vi "M-686 Test Panel.vi"() -> ()   [LabVIEW 2020]
uses:
  <vilib>/Instr/_visa.llb/VISA Configure Serial Port (Instr).vi
panel:
  in  "Wait for Reply":bool=TRUE
  out "Bool":bool
  out "Value":dbl
  out "Cmd Success":bool
  out "Connected":bool
  out "Waiting for Reply":bool
  out "Last Error":errorcluster
  out "Command History":string
  out "Reply":string
  in  "Command":string
  in  "Quit":bool
  in  "COM Port":refnum<visa-resource-name>="COM4"
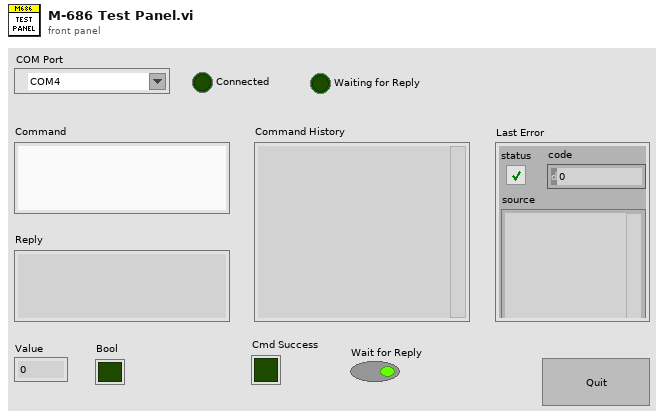
[diagram p1: front panel]
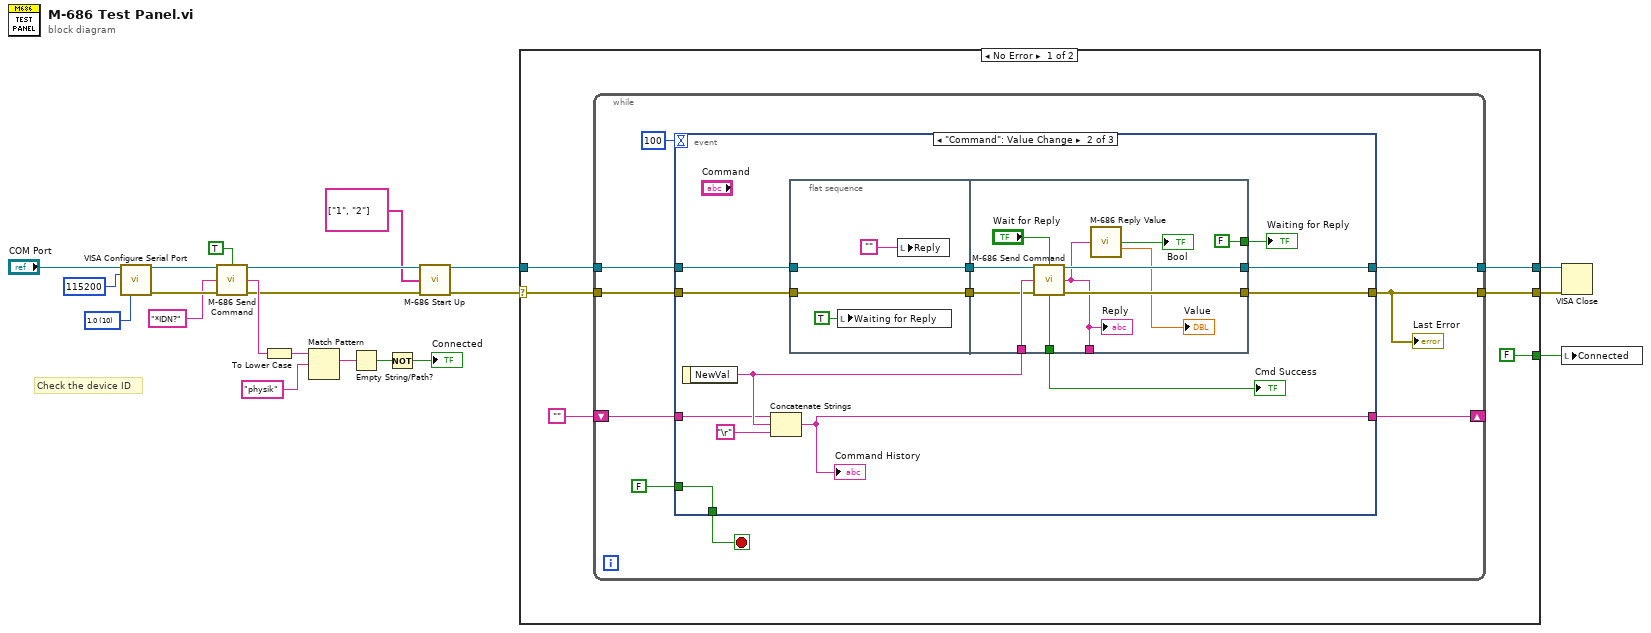
[diagram p0: block diagram]
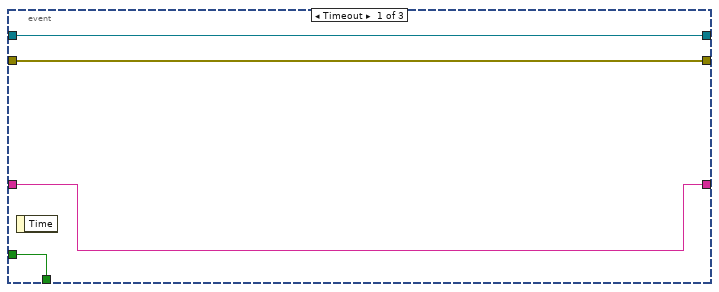
[diagram p2: hidden frame]
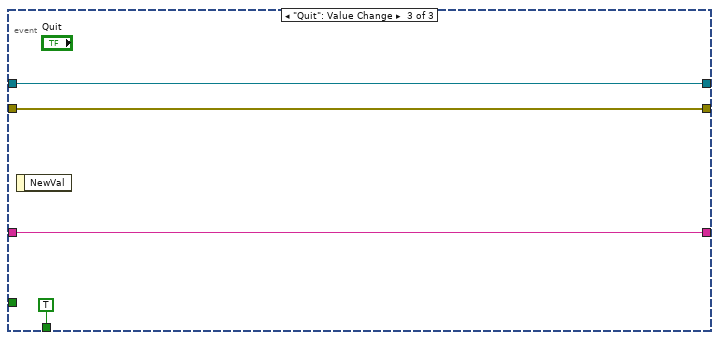
[diagram p3: hidden frame]
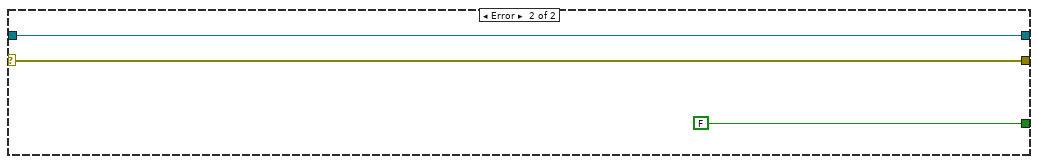
[diagram p4: hidden frame]
diagram:
  w18 = u16 10 items=["1.0"=10, "1.5"=15, "2.0"=20] ("stop bits (10: 1 bit)")
  # "Check the device ID"
  n1 = call-poly "VISA Configure Serial Port"("VISA resource name"="COM Port", "baud rate (9600)"=u32 115200, "stop bits (10: 1 bit)"=w18) -> ("VISA resource name out"=w16:refnum<visa-resource-name>, "error out"=w15:errorcluster)  [unwired: 11 in]
  n2 = call "M-686 Send Command.vi"("VISA Ref"=w16, "Wait for Reply (T)"=TRUE ("Wait for Reply?"), "Command"="*IDN?" ("string"), "Error In"=w15) -> ("VISA Ref Dup"=w5:refnum<visa-resource-name>, "Reply"=w11:string, "Error Out"=w4:errorcluster)  [unwired: 8 in, 1 out]
  n3 = To Lower Case(string=w11) -> (all lower case string=w13:string)
  n4 = Match Pattern(string=w13, regular expression="physik" ("string")) -> (match substring=w7:string)  [unwired: 1 in, 3 out]
  n5 = Empty String/Path?(string/path=w7) -> (empty?=w9:bool)
  n6 = Not(x=w9) -> (.not. x?=→"Connected":bool)
  n7 = call "M-686 Start Up.vi"("VISA Ref"=w5, "Axes Names"=string[] ["1", "2"], "Error In"=w4) -> ("VISA Ref Dup"=w3:refnum<visa-resource-name>, "Error Out"=w2:errorcluster)  [unwired: 11 in]
  n8 = case shown="No Error" w2 {
    selector: w2 -> [w26 w74]
    tunnel: w3 -> [w27 w75]
    tunnel: [w25 w75] -> w21
    tunnel: [w24 w74] -> w20
    tunnel: [FALSE FALSE] -> w19
    frame No Error {
      n9 = while {
        tunnel: w27 -> [w34]
        tunnel: w26 -> [w33]
        tunnel: [w32] -> w25
        tunnel: [w29] -> w24
        shift-right: [w30] -> _
        shift-left: "" -> [w31]
        stop <- w35 stop-if-true
        n10 = event shown="[1] \"Command\": Value Change" {
          selector: _ -> [_ _ _]
          dyn-events: _ -> [_ _ _]
          timeout: 100 -> [_ _ _]
          tunnel: FALSE -> [w40 w53 _]
          tunnel: [w40 w53 TRUE] -> w35
          tunnel: w34 -> [w38 w52 w72]
          tunnel: w33 -> [w37 w51 w71]
          tunnel: [w38 w47 w72] -> w32
          tunnel: [w37 w48 w71] -> w29
          tunnel: w31 -> [w39 w44 w69]
          tunnel: [w39 w43 w69] -> w30
          event Timeout {
            n11 = event-data() -> ()  [unwired: 1 in, 1 out]
          }
          event "Command": Value Change {
            n12 = event-data() -> ("NewVal"=w46:string)  [unwired: 1 in]
            n13 = Concatenate Strings(w44, w46, "\r") -> (w43:string)
            "Command History" <- w43
            n14 = flat-sequence {
              tunnel: w51 -> [w56]
              tunnel: w52 -> [w57]
              tunnel: [w57] -> w50
              tunnel: [w56] -> w49
              tunnel: w46 -> [w67]
              tunnel: w50 -> [w68]
              tunnel: w49 -> [w66]
              tunnel: [w65] -> w48
              tunnel: [w64] -> w47
              tunnel: [FALSE] -> w42
              tunnel: [w61] -> w41
              tunnel: [w58] -> _
              frame #0 {
                n15 = local write "Waiting for Reply"(TRUE ("Waiting for Cmd")) -> ()
                n16 = local write "Reply"("") -> ()
              }
              frame #1 {
                n17 = call "M-686 Send Command.vi"("VISA Ref"=w68, "Wait for Reply (T)"="Wait for Reply", "Command"=w67, "Error In"=w66) -> ("VISA Ref Dup"=w64:refnum<visa-resource-name>, "Reply"=w58:string, "Cmd Success"=w61:bool, "Error Out"=w65:errorcluster)  [unwired: 8 in]
                "Reply" <- w58
                n18 = call "M-686 Reply Value.vi"("Cmd Reply"=w58) -> ("Bool"=→"Bool":bool, "Value"=→"Value":dbl)  [unwired: 11 in, 2 out]
              }
            }
            "Waiting for Reply" <- w42
            "Cmd Success" <- w41
          }
          event "Quit": Value Change {
            n19 = event-data() -> ()  [unwired: 1 in, 1 out]
          }
        }
        "Last Error" <- w29
      }
    }
    frame Error {
    }
  }
  n20 = VISA Close(VISA resource name=w21, error in (no error)=w20) -> ()  [unwired: 1 out]
  n21 = local write "Connected"(w19) -> ()
